vi "FPGAController_v4_slow.vi"() -> ()   [LabVIEW 2013]
uses:
  <vilib>/Utility/miscctls.llb/LVPointTypeDef.ctl
  <userlib>/_OpenG.lib/file/file.llb/Strip Path Extension - Path__ogtk.vi
  <vilib>/FPGAPlugInAG/PXI-7954R/niLvFpga_Open_PXI-7954R.vi
  <userlib>/_OpenG.lib/comparison/comparison.llb/Boolean Changed__ogtk.vi
  <vilib>/addons/database/Connection.llb/Conn Execute.vi
  <vilib>/addons/database/Recordset.llb/Rec Fetch Recordset Data (R).vi
  <vilib>/addons/database/Recordset.llb/Rec Destroy - Connection.vi
  <userlib>/_OpenG.lib/comparison/comparison.llb/DBL Changed__ogtk.vi
  <vilib>/Utility/error.llb/Error Cluster From Error Code.vi
  <vilib>/rvi/errors/niLvFpgaAdjustHostInterfaceError.vi
  <vilib>/FPGAPlugInAG/PXI-7954R/niLvFpga_Close_PXI-7954R.vi
  <vilib>/rvi/interface/nirviOpenFPGA/nirviOpenFPGA.xnode
  FPGA Bitfiles/correlationwithf_FPGATarget_FPGAcodeslow_ywMU-DMuSi0.lvbitx
  <vilib>/addons/database/_DB Variant To Data/Database Variant To Data.xnode
  <vilib>/rvi/interface/nirviMethod/nirviMethod.xnode
  <vilib>/FPGA/interface/niFpgaViExecutionMode.ctl
  <vilib>/rvi/interface/nirviReadWriteControl/nirviReadWriteControl.xnode
  <vilib>/rvi/interface/nirviCloseFPGA/nirviCloseFPGA.xnode
  <vilib>/addons/database/NI_Database_API.lvlib
  NiFpgaLv.dll
panel:
  out "Time Betwee Shots":dbl
  out "Del Armed":bool
  in  "Lower Threshold":bool
  in  "Raise Threshold":bool
  out "Update Threshold":bool
  in  "Min. Time\nBetween Shots (s)":dbl
  in  "Rate Limiting":bool
  out "Armed":bool
  in  "Add Delay":bool
  in  "Delay Name":string
  in  "Delay Value":dbl=3.0 min=0.0
  in  "Delay Ring":dbl(ring)=3.15039 items=["Ablation Chamber"=6.45, "LEIL Chamber"=4.318, "Thid Detector"=3.15039, "Custom"=0.0]
  in  "Rearm Trigger":bool
  in  "One Shot Mode":bool
  out "Last Update:":timestamp
  out "Updating FPGA":bool
  out "Sensitivity":dbl
  out "error out":errorcluster
  out "Low Mass Limit":fxp<+,31,17>
  out "High Mass Limit":fxp<+,31,17>
  out "stopping":bool
  in  "Auto Threshold":bool
  out "Peletron (MV)":dbl=2.0
  out "High Mass (kg)":dbl=inf
  out "Low Mass (kg)":dbl
  out "High Charge Limit":i16
  out "Low Charge Limit":i16
  out "High velocity count":i32=210
  out "Low velocity count":i32=21000
  in  "stop":bool
  in  "Peak-Threshold Factor":dbl=2.0
  out "Low Charge Limit (fC)":dbl
  out "High Charge Limit (fC)":dbl=100.0
  out "High Velocity":dbl=100000.0
  out "Low Velocity":dbl=1000.0
  out "Filter 7 Peak":i32=7483
  out "Filter 6 Peak":i32=9863
  out "Filter 5 Peak":i32=13910
  out "Filter 4 Peak":i32=18191
  out "Filter 3 Peak":i32=46254
  out "Filter 2 Peak":i32=120664
  out "Filter 1 Peak":i32=295996
  in  "Filter7 Threshold":i32=-21165
  in  "Filter6 Threshold":i32=-29358
  in  "Filter5 Threshold":i32=-41730
  in  "Filter4 Threshold":i32=-54306
  in  "Filter3 Threshold":i32=-138762
  in  "Filter2 Threshold":i32=-361992
  in  "Filter1 Threshold":i32=-887988
  in  "Zero Peak Values":bool
  in  "Assign Threshold":bool
  in  "Run Mode":bool
  # "Settings"
  # "Dubugging"
  # "Independent Variable"
  # "Low Vel."
  # "High Vel."
  # "Low Q (fC)"
  # "High Q (fC)"
  # "Plate Control While Loop Counter"
  # "Low Mass (kg)"
  # "High Mass (kg)"
  # "Sens. (V/pC)"
  # "Peletron (MV)"
  # "Current Value of Running Average"
  # "Peak Threshold Factor"
  # "Delay Trigger"
  # "Dist. from 2nd Det. (m)"
  # "Name"
  # "Peak Values"
  # "Peak 1"
  # "Peak 2"
  # "Peak 3"
  # "Peak 4"
  # "Peak 5"
  # "Peak 6"
  # "Peak 7"
  # "Thresholds"
  # "Threshold 1"
  # "Threshold 2"
  # "Threshold 3"
  # "Threshold 4"
  # "Threshold 5"
  # "Threshold 6"
  # "Threshold 7"
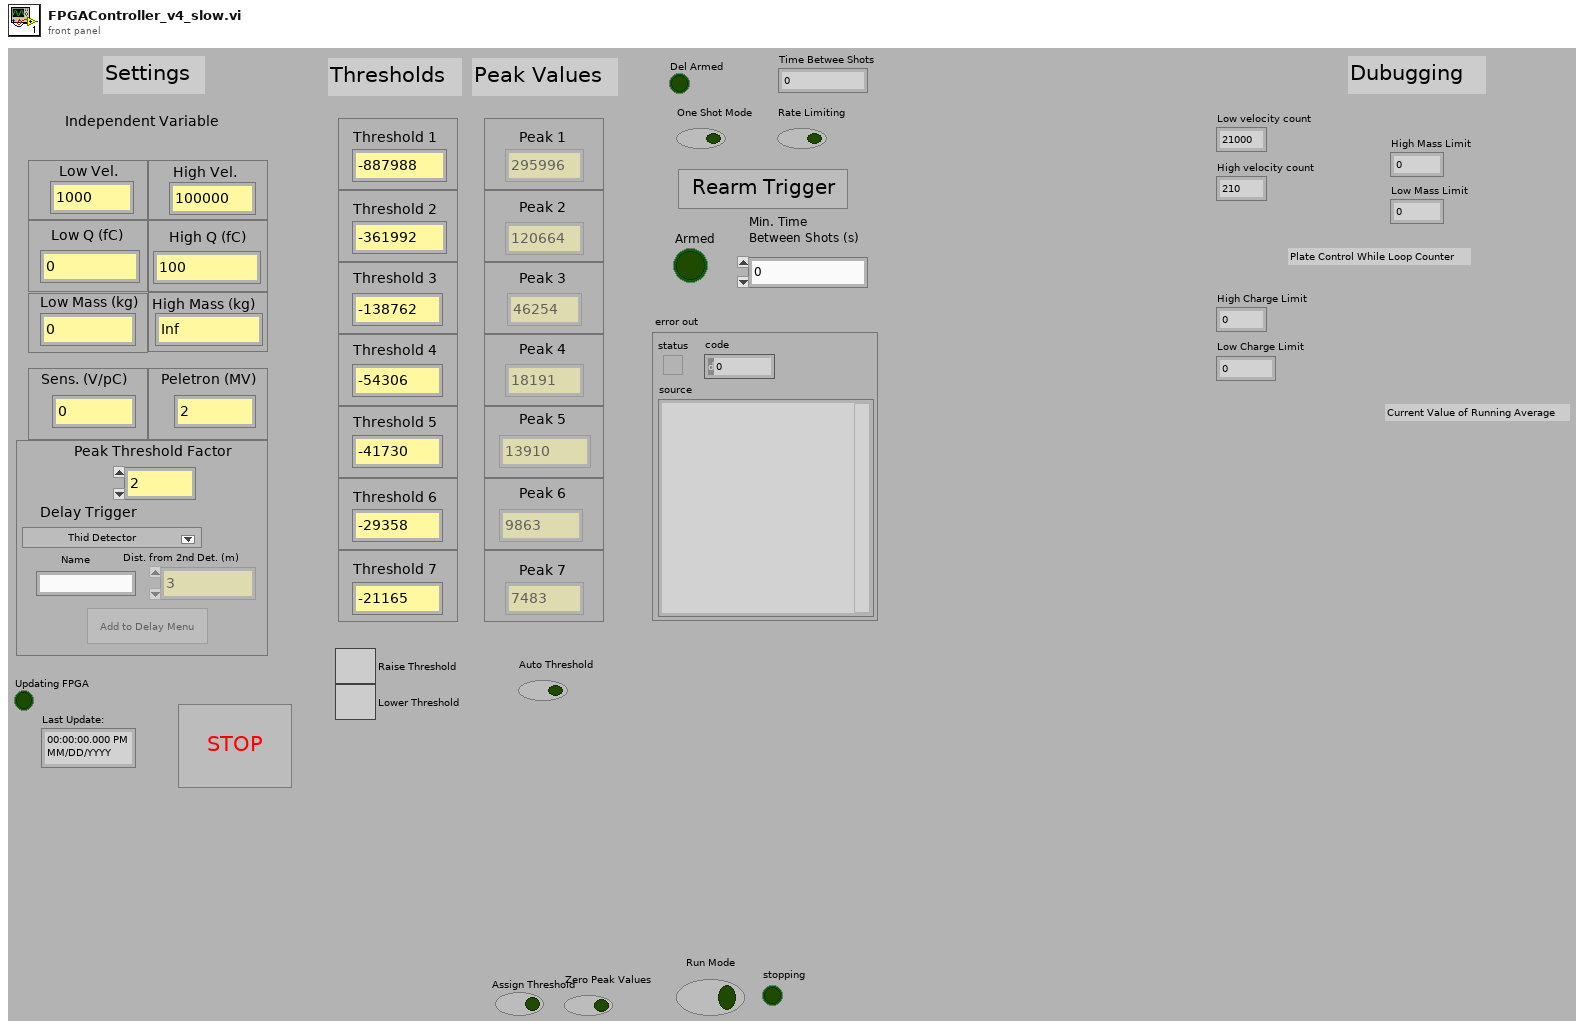
[diagram p1: front panel]
types:
  T1 = typedef "LVPointTypeDef.ctl" = cluster{"Horizontal":i16, "Vertical":i16}
  T2 = enum8{"Enabled", "Disabled", "Disabled and Grayed Out"}
  T3 = typedef "NI_Database_API.lvlib/Conn ObjectReference.ctl" = refnum<k1>
  T4 = cluster{"Filter 1 Peak":i32, "Filter 2 Peak":i32, "Filter 3 Peak":i32, "Filter 4 Peak":i32, "Filter 5 Peak":i32, "Filter 6 Peak":i32, "Filter 7 Peak":i32}
  T5 = typedef "NI_Database_API.lvlib/Rec ObjectReference.ctl" = refnum<k1>
  T6 = typedef "LVStringsAndValuesArrayTypeDef_DBL.ctl" = cluster{"String":string, "Value":dbl}[]
  T7 = cluster{"Numeric":dbl, "Numeric":dbl, "Numeric":dbl, "Numeric":dbl, "Numeric":dbl, "Numeric":dbl, dbl, dbl, "Value":dbl, fxp<+,16,7>, bool}
  T8 = cluster{"Low Velocity Count":i32, "High Velocity Count":i32, "Low Charge Limit (ADC ticks)":i16, "High Charge Limit (ADC ticks)":i16, "Low Mass (ADC*cycle^2)":i64, "High Mass (ADC*cycle^2)":i64, "Mult":fxp<+,16,7>, "Mult Use?":bool}
  T9 = cluster{"Filter 1 Detector 3 Correlation":i32, "Filter 2 Detector 3 Correlation":i32, "Filter 3 Detector 3 Correlation":i32, "Filter 4 Detector 3 Correlation":i32, "Filter 5 Detector 3 Correlation":i32, "Filter 6 Detector 3 Correlation":i32, "Filter 7 Detector 3 Correlation":i32}
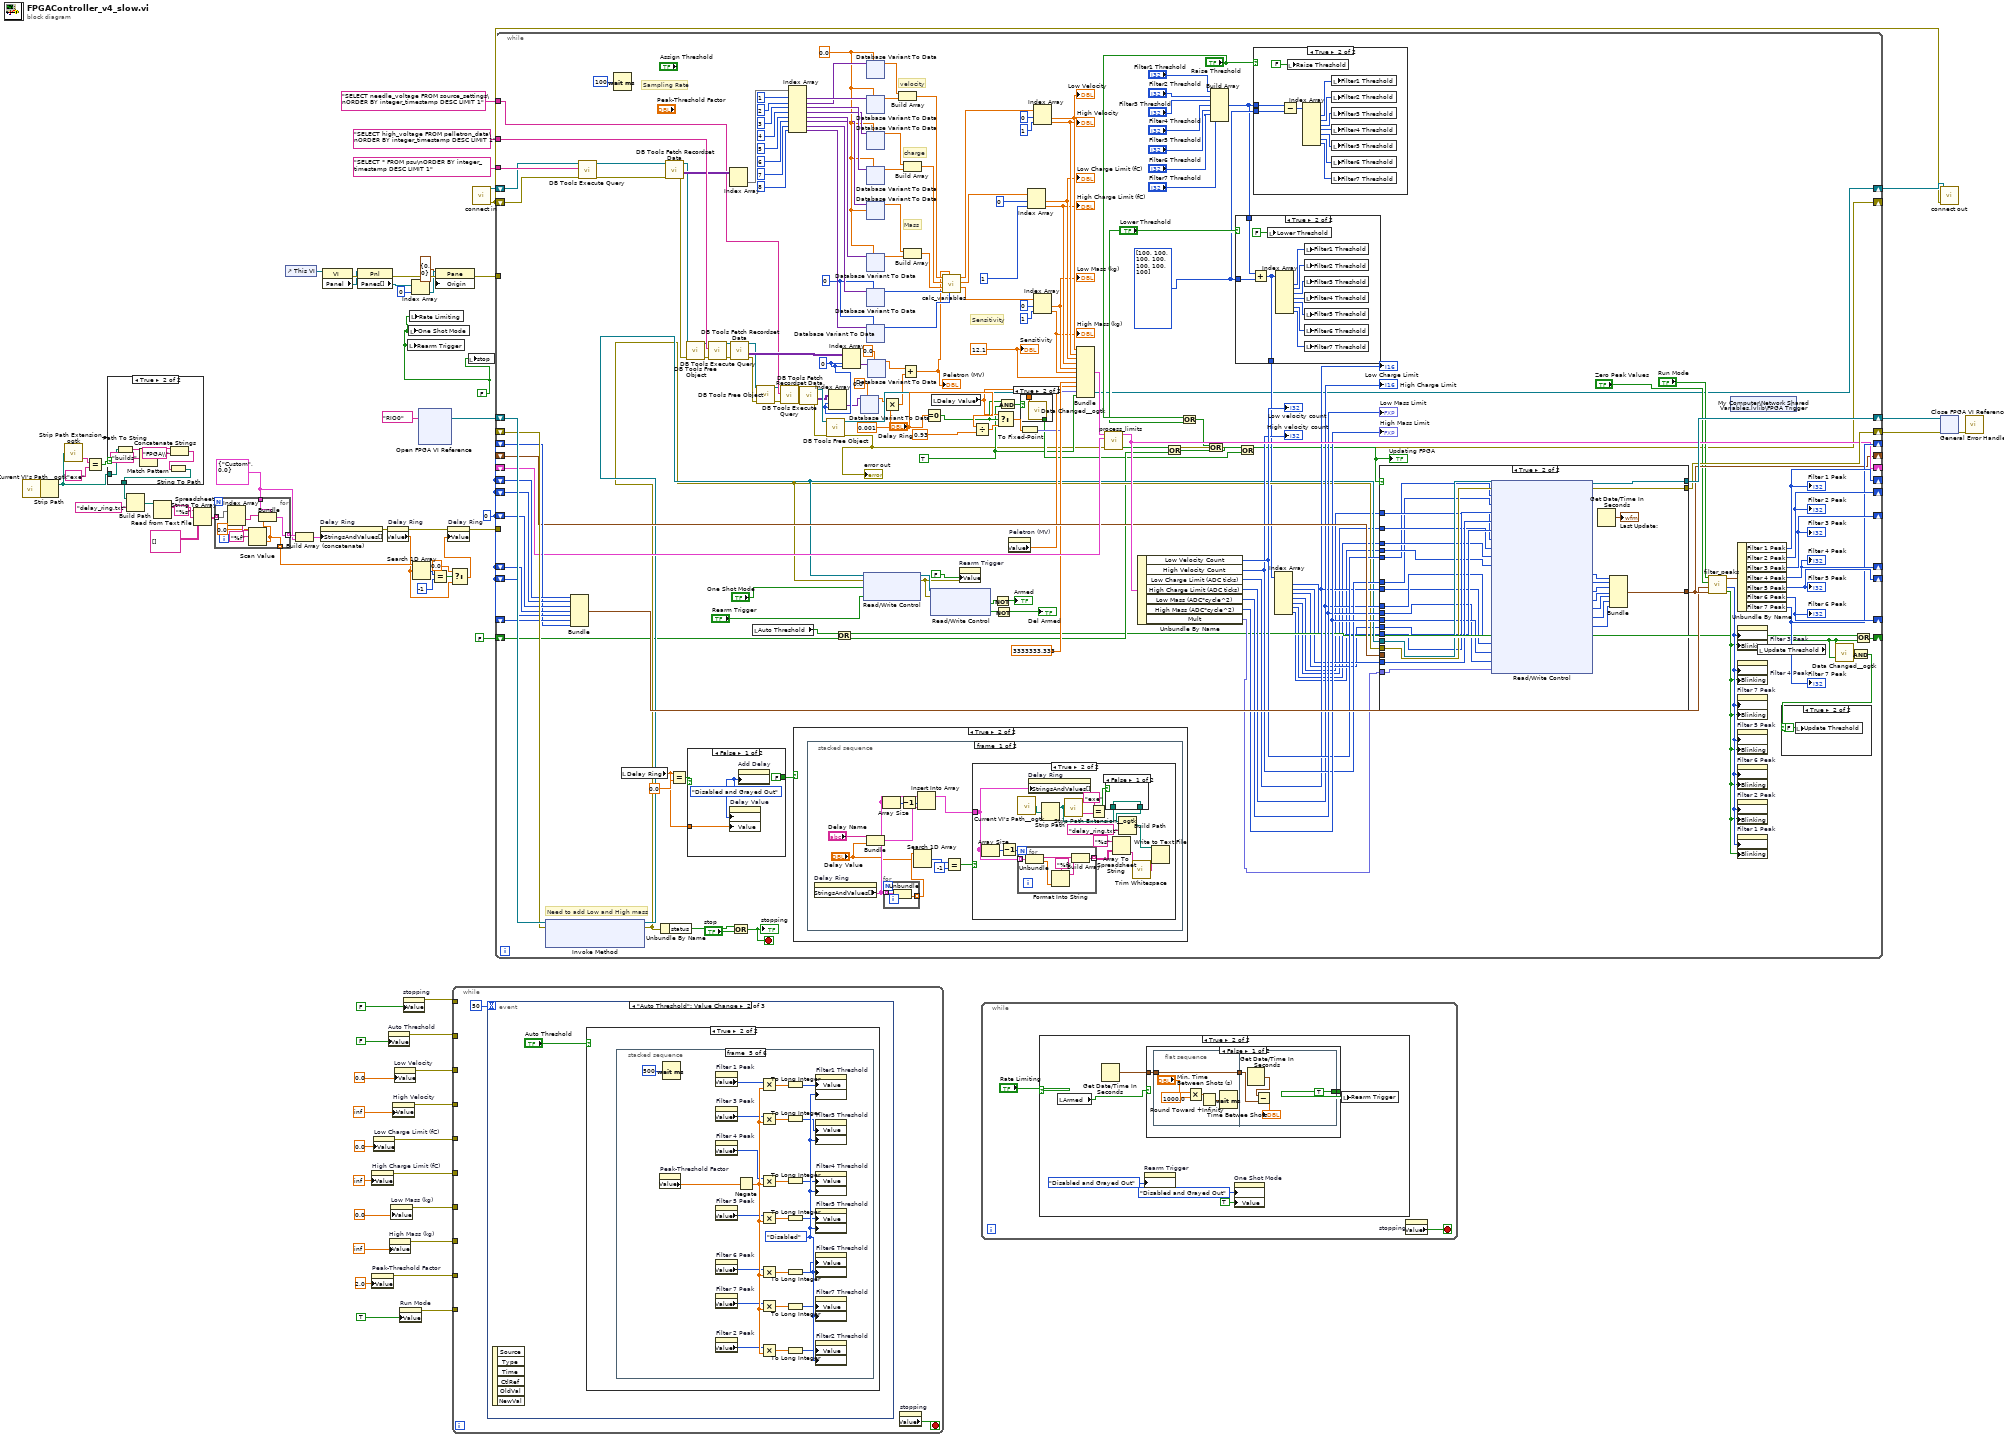
[diagram p0: block diagram]
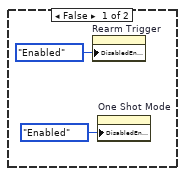
[diagram p3: hidden frame]
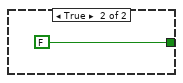
[diagram p4: hidden frame]
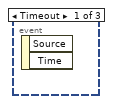
[diagram p5: hidden frame]
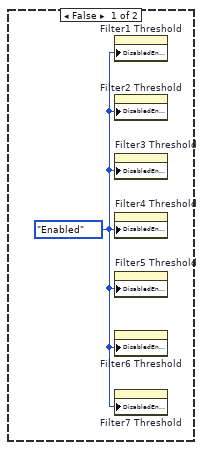
[diagram p6: hidden frame]
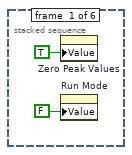
[diagram p7: hidden frame]
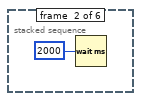
[diagram p8: hidden frame]
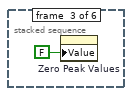
[diagram p9: hidden frame]
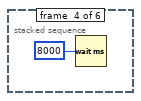
[diagram p10: hidden frame]
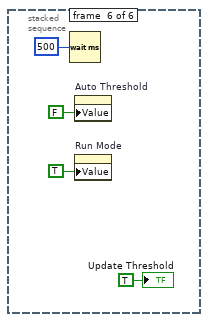
[diagram p11: hidden frame]
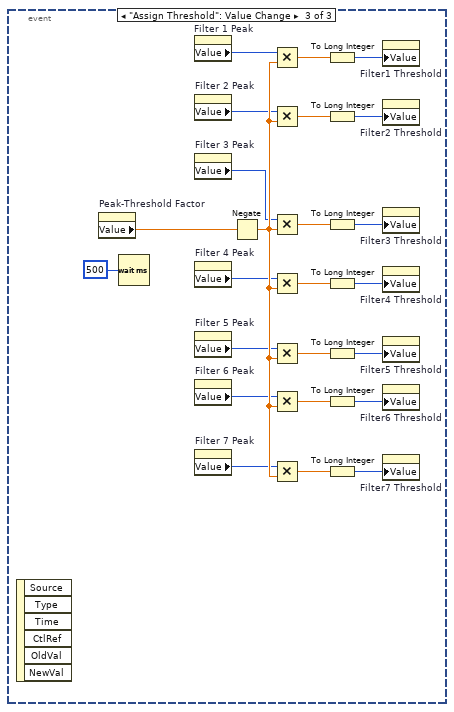
[diagram p12: hidden frame]
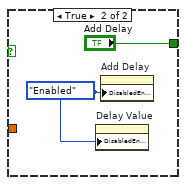
[diagram p17: hidden frame]
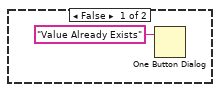
[diagram p19: hidden frame]
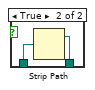
[diagram p20: hidden frame]
diagram:
  w18 = cluster{"String":string, "Value":dbl} {"String"="Custom", "Value"=0.0}
  w28 = FALSE
  w67 = 0
  n1 = call <userlib>:"Current VI's Path__ogtk.vi"() -> ("Current VI's Path (+ Relative)"=w27:path)  [unwired: 1 in]
  n2 = Strip Path(path=w27) -> (stripped path=w13:path)  [unwired: 1 out]
  n3 = call-poly <userlib>:"Strip Path Extension__ogtk.vi"("path"=w13) -> ("extension"=w17:string)  [unwired: 1 out]
  n4 = Equal?(x=w17, y="exe") -> (x = y?=w14:bool)
  n5 = case shown="True" w14 {
    tunnel: w13 -> [w69 w76]
    tunnel: [w69 w70] -> w12
    frame False {
    }
    frame True {
      n6 = Path To String(path=w76) -> (string=w75:string)
      n7 = Match Pattern(string=w75, regular expression="builds") -> (before substring=w73:string)  [unwired: 1 in, 3 out]
      n8 = Concatenate Strings(w73, "FPGA\\" ("string")) -> (w71:string)
      n9 = String To Path(string=w71) -> (path=w70:path)
    }
  }
  n10 = Build Path(base path=w12, name or relative path="delay_ring.txt") -> (appended path=w15:path)
  n11 = Read from Text File(file (use dialog)=w15) -> (text=w25:string)  [unwired: 3 in, 3 out]
  n12 = Spreadsheet String To Array(format string="%s", spreadsheet string=w25, array type (2D Dbl)=string[][] []) -> (array=w22:string[][])  [unwired: 1 in]
  n13 = for {
    tunnel: w22 -> [w84] mode=indexing
    tunnel: w18 -> [w82]
    tunnel: [w78] -> w19 mode=indexing
    tunnel: [w77] -> w11 mode=indexing
    n14 = Index Array(array=w84) -> (element #1=w83:string, element #2=w81:string)  [unwired: 2 in]
    n15 = Scan Value(string=w81, format string="%f", default (0 dbl)=0.0) -> (value=w77:dbl)  [unwired: 1 out]
    n16 = Bundle(cluster=w82, "String"=w83, "Value"=w77) -> (w78:cluster{"String":string, "Value":dbl})
  }
  n17 = control-ref of="This VI"() -> (w39:refnum<vi>)
  n18 = Build Array (concatenate)(w19, w18) -> (w21:cluster{"String":string, "Value":dbl}[])
  n19 = property on="Delay Ring" class="Ring (strict)"("StringsAndValues[]"=w21) -> (error out=w20:errorcluster)  [unwired: 2 in, 1 out]
  n20 = property class="VI"(reference=w39) -> (error out=w38:errorcluster, "Panel"=w37:refnum<vi>)  [unwired: 1 in, 1 out]
  n21 = property class="Pnl"(reference=w37, error in=w38) -> (error out=w36:errorcluster, "Panes[]"=w35:refnum<vi>[])  [unwired: 1 out]
  n22 = property on="High Charge Limit (fC)" class="DigNum (strict)"("Value"=inf ("High Charge Limit (fC)")) -> (error out=w54:errorcluster)  [unwired: 2 in, 1 out]
  n23 = property on="Peak-Threshold Factor" class="DigNum (strict)"("Value"=2.0 ("Peak-Threshold Factor")) -> (error out=w48:errorcluster)  [unwired: 2 in, 1 out]
  n24 = property on="Low Charge Limit (fC)" class="DigNum (strict)"("Value"=0.0 ("Low Charge Limit (fC)")) -> (error out=w56:errorcluster)  [unwired: 2 in, 1 out]
  n25 = property on="Delay Ring" class="Ring (strict)"(error in=w20) -> (error out=w10:errorcluster, "Value"=w4:dbl)  [unwired: 1 in, 1 out]
  n26 = property on="Auto Threshold" class="Bool (strict)"("Value"=FALSE ("Auto Threshold")) -> (error out=w62:errorcluster)  [unwired: 2 in, 1 out]
  n27 = property on="High Mass (kg)" class="DigNum (strict)"("Value"=inf ("High Mass (kg)")) -> (error out=w50:errorcluster)  [unwired: 2 in, 1 out]
  n28 = property on="Low Mass (kg)" class="DigNum (strict)"("Value"=0.0 ("Low Mass (kg)")) -> (error out=w52:errorcluster)  [unwired: 2 in, 1 out]
  n29 = property on="High Velocity" class="DigNum (strict)"("Value"=inf ("High Velocity")) -> (error out=w58:errorcluster)  [unwired: 2 in, 1 out]
  n30 = property on="Low Velocity" class="DigNum (strict)"("Value"=0.0 ("Low Velocity")) -> (error out=w60:errorcluster)  [unwired: 2 in, 1 out]
  n31 = property on="Run Mode" class="Bool (strict)"("Value"=TRUE ("Run Mode")) -> (error out=w46:errorcluster)  [unwired: 2 in, 1 out]
  n32 = property on="stopping" class="Bool (strict)"("Value"=FALSE ("stopping")) -> (error out=w64:errorcluster)  [unwired: 2 in, 1 out]
  n33 = local write "Rearm Trigger"(w28) -> ()
  n34 = local write "One Shot Mode"(w28) -> ()
  n35 = local write "Rate Limiting"(w28) -> ()
  n36 = Index Array(array=w35, index=0) -> (element=w33:refnum<vi>)
  n37 = Search 1D Array(1D array=w11, element=w4) -> (index of element=w8:i32)  [unwired: 1 in]
  n38 = xnode "Open FPGA VI Reference"("resource name"=tag "RIO0") -> ("FPGA VI Reference Out"=w30:refnum<k20>)  [unwired: 1 in, 1 out]
  n39 = Equal?(x=w8, y=-1) -> (x = y?=w6:bool)
  n40 = property class="Pane"(reference=w33, error in=w36, "Origin"=T1 {"Horizontal"=0, "Vertical"=0}) -> (error out=w31:errorcluster)  [unwired: 1 out]
  n41 = Select(t=0.0, s=w6, f=w4) -> (s? t:f=w5:dbl)
  n42 = property on="Delay Ring" class="Ring (strict)"(error in=w10, "Value"=w5) -> (error out=w9:errorcluster)  [unwired: 1 in, 1 out]
  n43 = while {
    tunnel: w64 -> [_]
    tunnel: w62 -> [_]
    tunnel: w60 -> [_]
    tunnel: w58 -> [_]
    tunnel: w56 -> [_]
    tunnel: w54 -> [_]
    tunnel: w52 -> [_]
    tunnel: w50 -> [_]
    tunnel: w48 -> [_]
    tunnel: w46 -> [_]
    stop <- w86 stop-if-true
    n44 = event shown="[1] \"Auto Threshold\": Value Change" {
      selector: _ -> [_ _ _]
      dyn-events: _ -> [_ _ _]
      timeout: 50 -> [_ _ _]
      event Timeout {
        n45 = event-data() -> ()  [unwired: 1 in, 2 out]
      }
      event "Auto Threshold": Value Change {
        n46 = event-data() -> ()  [unwired: 1 in, 6 out]
        n47 = case shown="True" "Auto Threshold" {
          frame False {
            w88 = T2."Enabled" ("Disabled")
            n48 = property on="Filter1 Threshold" class="DigNum (strict)"("DisabledEnum"=w88) -> ()  [unwired: 2 in, 2 out]
            n49 = property on="Filter2 Threshold" class="DigNum (strict)"("DisabledEnum"=w88) -> ()  [unwired: 2 in, 2 out]
            n50 = property on="Filter3 Threshold" class="DigNum (strict)"("DisabledEnum"=w88) -> ()  [unwired: 2 in, 2 out]
            n51 = property on="Filter4 Threshold" class="DigNum (strict)"("DisabledEnum"=w88) -> ()  [unwired: 2 in, 2 out]
            n52 = property on="Filter5 Threshold" class="DigNum (strict)"("DisabledEnum"=w88) -> ()  [unwired: 2 in, 2 out]
            n53 = property on="Filter6 Threshold" class="DigNum (strict)"("DisabledEnum"=w88) -> ()  [unwired: 2 in, 2 out]
            n54 = property on="Filter7 Threshold" class="DigNum (strict)"("DisabledEnum"=w88) -> ()  [unwired: 2 in, 2 out]
          }
          frame True {
            n55 = stacked-sequence {
              frame #0 {
                n56 = property on="Zero Peak Values" class="Bool (strict)"("Value"=TRUE ("Zero Peak Values")) -> ()  [unwired: 2 in, 2 out]
                n57 = property on="Run Mode" class="Bool (strict)"("Value"=FALSE ("Run Mode")) -> ()  [unwired: 2 in, 2 out]
              }
              frame #1 {
                n58 = Wait (ms)(milliseconds to wait=u32 2000) -> ()  [unwired: 1 out]
              }
              frame #2 {
                n59 = property on="Zero Peak Values" class="Bool (strict)"("Value"=FALSE ("Zero Peak Values")) -> ()  [unwired: 2 in, 2 out]
              }
              frame #3 {
                n60 = Wait (ms)(milliseconds to wait=u32 8000) -> ()  [unwired: 1 out]
              }
              frame #4 {
                w118 = T2."Disabled" ("Disabled")
                n61 = property on="Peak-Threshold Factor" class="DigNum (strict)"() -> ("Value"=w103:dbl)  [unwired: 2 in, 2 out]
                n62 = Wait (ms)(milliseconds to wait=u32 500) -> ()  [unwired: 1 out]
                n63 = property on="Filter 1 Peak" class="DigNum (strict)"() -> ("Value"=w101:i32)  [unwired: 2 in, 2 out]
                n64 = property on="Filter 3 Peak" class="DigNum (strict)"() -> ("Value"=w99:i32)  [unwired: 2 in, 2 out]
                n65 = property on="Filter 4 Peak" class="DigNum (strict)"() -> ("Value"=w98:i32)  [unwired: 2 in, 2 out]
                n66 = property on="Filter 5 Peak" class="DigNum (strict)"() -> ("Value"=w97:i32)  [unwired: 2 in, 2 out]
                n67 = property on="Filter 6 Peak" class="DigNum (strict)"() -> ("Value"=w96:i32)  [unwired: 2 in, 2 out]
                n68 = property on="Filter 7 Peak" class="DigNum (strict)"() -> ("Value"=w95:i32)  [unwired: 2 in, 2 out]
                n69 = property on="Filter 2 Peak" class="DigNum (strict)"() -> ("Value"=w100:i32)  [unwired: 2 in, 2 out]
                n70 = Negate(x=w103) -> (-x=w102:dbl)
                n71 = Multiply(x=w101, y=w102) -> (x*y=w117:dbl)
                n72 = Multiply(x=w99, y=w102) -> (x*y=w113:dbl)
                n73 = Multiply(x=w98, y=w102) -> (x*y=w111:dbl)
                n74 = Multiply(x=w97, y=w102) -> (x*y=w109:dbl)
                n75 = Multiply(x=w96, y=w102) -> (x*y=w107:dbl)
                n76 = Multiply(x=w95, y=w102) -> (x*y=w105:dbl)
                n77 = Multiply(x=w100, y=w102) -> (x*y=w115:dbl)
                n78 = To Long Integer(number=w117) -> (32bit integer=w116:i32)
                n79 = To Long Integer(number=w113) -> (32bit integer=w112:i32)
                n80 = To Long Integer(number=w111) -> (32bit integer=w110:i32)
                n81 = To Long Integer(number=w109) -> (32bit integer=w108:i32)
                n82 = To Long Integer(number=w107) -> (32bit integer=w106:i32)
                n83 = To Long Integer(number=w105) -> (32bit integer=w104:i32)
                n84 = To Long Integer(number=w115) -> (32bit integer=w114:i32)
                n85 = property on="Filter1 Threshold" class="DigNum (strict)"("Value"=w116, "DisabledEnum"=w118) -> ()  [unwired: 2 in, 2 out]
                n86 = property on="Filter3 Threshold" class="DigNum (strict)"("Value"=w112, "DisabledEnum"=w118) -> ()  [unwired: 2 in, 2 out]
                n87 = property on="Filter4 Threshold" class="DigNum (strict)"("Value"=w110, "DisabledEnum"=w118) -> ()  [unwired: 2 in, 2 out]
                n88 = property on="Filter5 Threshold" class="DigNum (strict)"("Value"=w108, "DisabledEnum"=w118) -> ()  [unwired: 2 in, 2 out]
                n89 = property on="Filter6 Threshold" class="DigNum (strict)"("Value"=w106, "DisabledEnum"=w118) -> ()  [unwired: 2 in, 2 out]
                n90 = property on="Filter7 Threshold" class="DigNum (strict)"("Value"=w104, "DisabledEnum"=w118) -> ()  [unwired: 2 in, 2 out]
                n91 = property on="Filter2 Threshold" class="DigNum (strict)"("Value"=w114, "DisabledEnum"=w118) -> ()  [unwired: 2 in, 2 out]
              }
              frame #5 {
                n92 = Wait (ms)(milliseconds to wait=u32 500) -> ()  [unwired: 1 out]
                n93 = property on="Auto Threshold" class="Bool (strict)"("Value"=FALSE ("Auto Threshold")) -> ()  [unwired: 2 in, 2 out]
                n94 = property on="Run Mode" class="Bool (strict)"("Value"=TRUE ("Run Mode")) -> ()  [unwired: 2 in, 2 out]
                "Update Threshold" <- TRUE ("Update Threshold")
              }
            }
          }
        }
      }
      event "Assign Threshold": Value Change {
        n95 = event-data() -> ()  [unwired: 1 in, 6 out]
        n96 = property on="Peak-Threshold Factor" class="DigNum (strict)"() -> ("Value"=w137:dbl)  [unwired: 2 in, 2 out]
        n97 = Wait (ms)(milliseconds to wait=u32 500) -> ()  [unwired: 1 out]
        n98 = property on="Filter 1 Peak" class="DigNum (strict)"() -> ("Value"=w136:i32)  [unwired: 2 in, 2 out]
        n99 = property on="Filter 2 Peak" class="DigNum (strict)"() -> ("Value"=w135:i32)  [unwired: 2 in, 2 out]
        n100 = property on="Filter 3 Peak" class="DigNum (strict)"() -> ("Value"=w134:i32)  [unwired: 2 in, 2 out]
        n101 = property on="Filter 4 Peak" class="DigNum (strict)"() -> ("Value"=w133:i32)  [unwired: 2 in, 2 out]
        n102 = property on="Filter 5 Peak" class="DigNum (strict)"() -> ("Value"=w132:i32)  [unwired: 2 in, 2 out]
        n103 = property on="Filter 6 Peak" class="DigNum (strict)"() -> ("Value"=w131:i32)  [unwired: 2 in, 2 out]
        n104 = property on="Filter 7 Peak" class="DigNum (strict)"() -> ("Value"=w130:i32)  [unwired: 2 in, 2 out]
        n105 = Negate(x=w137) -> (-x=w139:dbl)
        n106 = Multiply(x=w136, y=w139) -> (x*y=w146:dbl)
        n107 = Multiply(x=w135, y=w139) -> (x*y=w144:dbl)
        n108 = Multiply(x=w134, y=w139) -> (x*y=w143:dbl)
        n109 = Multiply(x=w133, y=w139) -> (x*y=w142:dbl)
        n110 = Multiply(x=w132, y=w139) -> (x*y=w141:dbl)
        n111 = Multiply(x=w131, y=w139) -> (x*y=w140:dbl)
        n112 = Multiply(x=w130, y=w139) -> (x*y=w145:dbl)
        n113 = To Long Integer(number=w146) -> (32bit integer=w129:i32)
        n114 = To Long Integer(number=w144) -> (32bit integer=w128:i32)
        n115 = To Long Integer(number=w143) -> (32bit integer=w127:i32)
        n116 = To Long Integer(number=w142) -> (32bit integer=w126:i32)
        n117 = To Long Integer(number=w141) -> (32bit integer=w125:i32)
        n118 = To Long Integer(number=w140) -> (32bit integer=w124:i32)
        n119 = To Long Integer(number=w145) -> (32bit integer=w123:i32)
        n120 = property on="Filter1 Threshold" class="DigNum (strict)"("Value"=w129) -> ()  [unwired: 2 in, 2 out]
        n121 = property on="Filter2 Threshold" class="DigNum (strict)"("Value"=w128) -> ()  [unwired: 2 in, 2 out]
        n122 = property on="Filter3 Threshold" class="DigNum (strict)"("Value"=w127) -> ()  [unwired: 2 in, 2 out]
        n123 = property on="Filter4 Threshold" class="DigNum (strict)"("Value"=w126) -> ()  [unwired: 2 in, 2 out]
        n124 = property on="Filter5 Threshold" class="DigNum (strict)"("Value"=w125) -> ()  [unwired: 2 in, 2 out]
        n125 = property on="Filter6 Threshold" class="DigNum (strict)"("Value"=w124) -> ()  [unwired: 2 in, 2 out]
        n126 = property on="Filter7 Threshold" class="DigNum (strict)"("Value"=w123) -> ()  [unwired: 2 in, 2 out]
      }
    }
    n127 = property on="stopping" class="Bool (strict)"() -> ("Value"=w86:bool)  [unwired: 2 in, 2 out]
  }
  n128 = local write "stop"(w28) -> ()
  n129 = call "connect in.vi"() -> ("error out"=w40:errorcluster, "Database Connection"=w41:T3)  [unwired: 7 in, 1 out]
  n130 = while {
    shift-right: [w322] -> w66
    shift-left: w30 -> [w326]
    shift-right: [w321] -> w65
    shift-left: _ -> [w325]
    shift-right: [w317] -> _
    shift-left: w67 -> [w310]
    shift-right: [w316] -> _
    shift-left: w67 -> [w309]
    shift-right: [w315] -> _
    shift-left: w67 -> [w308]
    shift-right: [w314] -> _
    shift-left: w67 -> [w307]
    shift-right: [w313] -> _
    shift-left: w67 -> [w306]
    shift-right: [w319] -> _
    shift-left: w67 -> [w312]
    shift-right: [w318] -> _
    shift-left: w67 -> [w311]
    tunnel: "SELECT * FROM psu\nORDER BY integer_timestamp DESC LIMIT 1" ("SQL query") -> [w305]
    tunnel: "SELECT high_voltage FROM pelletron_data\nORDER BY integer_timestamp DESC LIMIT 1" ("SQL query") -> [w304]
    shift-right: [w156] -> w42
    shift-left: w41 -> [w303]
    shift-right: [w157] -> _
    shift-left: w40 -> [w302]
    shift-right: [w301] -> _
    shift-left: _ -> [w300]
    shift-right: [w298] -> _
    shift-left: _ -> [w299]
    tunnel: w31 -> [_]
    tunnel: w9 -> [_]
    shift-right: [w203] -> _
    shift-left: FALSE -> [w206]
    tunnel: "SELECT needle_voltage FROM source_settings\nORDER BY integer_timestamp DESC LIMIT 1" ("SQL query") -> [w164]
    stop <- w320 stop-if-true
    w166 = i32[] [100, 100, 100, 100, 100, 100, 100]
    w169 = TRUE
    w154 = 0 ("index (row)")
    w262 = i8 0
    w263 = 0.0
    w229 = 12.1
    # "charge"
    # "Mass"
    # "velocity"
    # "Sensitivity"
    # "Sampling Rate"
    # "Need to add Low and High mass"
    n131 = xnode "Invoke Method"("FPGA VI Reference In"=w326, "error in"=w325) -> ("FPGA VI Reference Out"=w223:refnum<k20>, "error out"=w222:errorcluster)  [unwired: 1 out]
    n132 = Bundle("Filter 1 Peak"=w312, "Filter 2 Peak"=w311, "Filter 3 Peak"=w310, "Filter 4 Peak"=w309, "Filter 5 Peak"=w308, "Filter 6 Peak"=w307, "Filter 7 Peak"=w306) -> (w294:T4)  [unwired: 1 in]
    n133 = call-poly <vilib>:"DB Tools Execute Query.vi"("error in (no error)"=w302, "SQL query"=w305, "connection reference"=w303) -> ("error out"=w282:errorcluster, "recordset reference"=w283:T5)  [unwired: 5 in]
    n134 = Wait (ms)(milliseconds to wait=u32 100) -> ()  [unwired: 1 out]
    n135 = local read "Delay Ring"() -> (w207:dbl)
    n136 = Unbundle By Name(w222) -> ("status"=w324:bool)
    n137 = call-poly <vilib>:"DB Tools Fetch Recordset Data.vi"("error in (no error)"=w282, "recordset reference"=w283) -> ("error out"=w260:errorcluster, "recordset data"=w273:variant[][], "recordset reference out"=w261:T5)  [unwired: 3 in]
    n138 = Equal?(x=w207, y=0.0) -> (x = y?=w208:bool)
    n139 = call-poly <vilib>:"DB Tools Free Object.vi"("error in (no error)"=w260, "recordset reference"=w261) -> ("error out"=w258:errorcluster, "connection reference"=w259:T3)  [unwired: 8 in]
    n140 = case shown="False" w208 {
      tunnel: [FALSE ("Add Delay") "Add Delay"] -> w226
      tunnel: w207 -> [w387 _]
      frame False {
        w388 = T2."Disabled and Grayed Out" ("Disabled")
        n141 = property on="Delay Value" class="DigNum (strict)"("DisabledEnum"=w388, "Value"=w387) -> ()  [unwired: 2 in, 2 out]
        n142 = property on="Add Delay" class="Bool (strict)"("DisabledEnum"=w388) -> ()  [unwired: 2 in, 2 out]
      }
      frame True {
        w389 = T2."Enabled" ("Disabled")
        n143 = property on="Delay Value" class="DigNum (strict)"("DisabledEnum"=w389) -> ()  [unwired: 2 in, 2 out]
        n144 = property on="Add Delay" class="Bool (strict)"("DisabledEnum"=w389) -> ()  [unwired: 2 in, 2 out]
      }
    }
    n145 = call-poly <vilib>:"DB Tools Execute Query.vi"("error in (no error)"=w258, "SQL query"=w304, "connection reference"=w259) -> ("error out"=w256:errorcluster, "recordset reference"=w257:T5)  [unwired: 5 in]
    n146 = Index Array(array=w273) -> (element=w272:variant[])  [unwired: 2 in]
    n147 = call-poly <vilib>:"DB Tools Fetch Recordset Data.vi"("error in (no error)"=w256, "recordset reference"=w257) -> ("error out"=w230:errorcluster, "recordset data"=w255:variant[][], "recordset reference out"=w231:T5)  [unwired: 3 in]
    n148 = Or(x=w324, y="stop") -> (x .or. y?=w320:bool)
    "stopping" <- w320
    n149 = local read "Auto Threshold"() -> (w204:bool)
    n150 = call-poly <vilib>:"DB Tools Free Object.vi"("error in (no error)"=w230, "recordset reference"=w231) -> ("error out"=w162:errorcluster, "connection reference"=w163:T3)  [unwired: 8 in]
    n151 = call-poly <vilib>:"DB Tools Execute Query.vi"("error in (no error)"=w162, "SQL query"=w164, "connection reference"=w163) -> ("error out"=w160:errorcluster, "recordset reference"=w161:T5)  [unwired: 5 in]
    n152 = Index Array(array=w272, index #1=1 ("index"), index #2=2 ("index"), index #3=3 ("index"), index #4=4 ("index"), index #5=5 ("index"), index #6=6 ("index"), index #7=7 ("index"), index #8=8 ("index")) -> (element #1=w271:variant, element #2=w270:variant, element #3=w269:variant, element #4=w268:variant, element #5=w267:variant, element #6=w266:variant, element #7=w265:variant, element #8=w264:variant)
    n153 = case shown="True" w226 {
      frame False {
      }
      frame True {
        n154 = stacked-sequence {
          frame #0 {
            n155 = property on="Delay Ring" class="Ring (strict)"() -> ("StringsAndValues[]"=w393:T6)  [unwired: 2 in, 2 out]
            n156 = Bundle("Delay Name"="Delay Name", "Delay Value"="Delay Value") -> (w398:cluster{"Delay Name":string, "Delay Value":dbl})  [unwired: 1 in]
            n157 = Array Size(array=w393) -> (size(s)=w396:i32)
            n158 = for {
              tunnel: w393 -> [w403] mode=indexing
              tunnel: [w402] -> w392 mode=indexing
              n159 = Unbundle(w403) -> ("Value"=w402:dbl)  [unwired: 1 out]
            }
            n160 = Decrement(x=w396) -> (x-1=w395:i32)
            n161 = Search 1D Array(1D array=w392, element="Delay Value") -> (index of element=w400:i32)  [unwired: 1 in]
            n162 = Insert Into Array(array=w393, index=w395, new element=w398) -> (w397:T6)
            n163 = Equal?(x=w400, y=-1) -> (x = y?=w394:bool)
            n164 = case shown="True" w394 {
              tunnel: w397 -> [_ w412]
              frame False {
                n165 = One Button Dialog(message="Value Already Exists") -> ()  [unwired: 1 in, 1 out]
              }
              frame True {
                n166 = Array Size(array=w412) -> (size(s)=w414:i32)
                n167 = Decrement(x=w414) -> (x-1=w413:i32)
                n168 = call <userlib>:"Current VI's Path__ogtk.vi"() -> ("Current VI's Path (+ Relative)"=w418:path)  [unwired: 1 in]
                n169 = for {
                  N: w413 -> [_]
                  tunnel: w412 -> [w428] mode=indexing
                  tunnel: [w423] -> w415 mode=indexing
                  n170 = Unbundle(w428) -> ("String"=w424:string, "Value"=w427:dbl)
                  n171 = Format Into String(format string="%f", w427) -> (resulting string=w425:string)  [unwired: 2 in, 1 out]
                  n172 = Build Array(w424, w425) -> (w423:string[])
                }
                n173 = property on="Delay Ring" class="Ring (strict)"("StringsAndValues[]"=w412) -> ()  [unwired: 2 in, 2 out]
                n174 = Strip Path(path=w418) -> (stripped path=w406:path)  [unwired: 1 out]
                n175 = call-poly <userlib>:"Strip Path Extension__ogtk.vi"("path"=w406) -> ("extension"=w409:string)  [unwired: 1 out]
                n176 = Equal?(x="exe", y=w409) -> (x = y?=w407:bool)
                n177 = case shown="False" w407 {
                  tunnel: w406 -> [w420 w422]
                  tunnel: [w420 w421] -> w405
                  frame False {
                  }
                  frame True {
                    n178 = Strip Path(path=w422) -> (stripped path=w421:path)  [unwired: 1 out]
                  }
                }
                n179 = Array To Spreadsheet String(array=w415, 3:"%s" ("format string")) -> (spreadsheet string=w411:string)  [unwired: 1 in]
                n180 = Build Path(base path=w405, name or relative path="delay_ring.txt") -> (appended path=w416:path)
                n181 = call <vilib>:"Trim Whitespace.vi"("string"=w411) -> ("trimmed string"=w410:string)  [unwired: 1 in]
                n182 = Write to Text File(file (use dialog)=w416, text=w410) -> ()  [unwired: 2 in, 3 out]
              }
            }
          }
          frame #1 {
            n183 = property on="Add Delay" class="Bool (strict)"("Value"=FALSE ("Add Delay")) -> ()  [unwired: 2 in, 2 out]
          }
        }
      }
    }
    n184 = call-poly <vilib>:"DB Tools Fetch Recordset Data.vi"("error in (no error)"=w160, "recordset reference"=w161) -> ("error out"=w158:errorcluster, "recordset data"=w155:variant[][], "recordset reference out"=w159:T5)  [unwired: 3 in]
    n185 = call-poly <vilib>:"DB Tools Free Object.vi"("error in (no error)"=w158, "recordset reference"=w159) -> ("error out"=w157:errorcluster, "connection reference"=w156:T3)  [unwired: 8 in]
    "error out" <- w157
    n186 = Index Array(array=w155, index (row)=w154, index (col)=w154) -> (element=w153:variant)
    n187 = Or(x=w204, y=w206) -> (x .or. y?=w205:bool)
    n188 = Index Array(array=w255, index (row)=w154, index (col)=w154) -> (element=w254:variant)
    n189 = xnode "Database Variant To Data"("database variant"=w153, "type"=0.0) -> ("data"=w151:dbl)  [unwired: 1 in, 1 out]
    n190 = xnode "Read/Write Control"("FPGA VI Reference In"=w223, "error in"=w222, "One Shot"="One Shot Mode", "Reset One Shot"="Rearm Trigger") -> ("FPGA VI Reference Out"=w216:refnum<k20>, "error out"=w215:errorcluster)
    n191 = xnode "Database Variant To Data"("database variant"=w270, "type"=w263) -> ("data"=w179:dbl)  [unwired: 1 in, 1 out]
    n192 = xnode "Database Variant To Data"("database variant"=w271, "type"=w263) -> ("data"=w180:dbl)  [unwired: 1 in, 1 out]
    n193 = xnode "Database Variant To Data"("database variant"=w268, "type"=w263) -> ("data"=w178:dbl)  [unwired: 1 in, 1 out]
    n194 = xnode "Database Variant To Data"("database variant"=w269, "type"=w263) -> ("data"=w177:dbl)  [unwired: 1 in, 1 out]
    n195 = xnode "Database Variant To Data"("database variant"=w266, "type"=w263) -> ("data"=w176:dbl)  [unwired: 1 in, 1 out]
    n196 = xnode "Database Variant To Data"("database variant"=w267, "type"=w263) -> ("data"=w175:dbl)  [unwired: 1 in, 1 out]
    n197 = xnode "Database Variant To Data"("database variant"=w265, "type"=w262) -> ("data"=w248:i8)  [unwired: 1 in, 1 out]
    n198 = xnode "Database Variant To Data"("database variant"=w264, "type"=w262) -> ("data"=w247:i8)  [unwired: 1 in, 1 out]
    n199 = xnode "Database Variant To Data"("database variant"=w254, "type"=0.0) -> ("data"=w149:dbl)  [unwired: 1 in, 1 out]
    n200 = Multiply(x=w151, y=0.001) -> (x*y=w148:dbl)
    n201 = Build Array(w179, w180) -> (w251:dbl[])
    n202 = Add(x=w149, y=w148) -> (x+y=w147:dbl)
    "Peletron (MV)" <- w147
    n203 = Build Array(w178, w177) -> (w250:dbl[])
    n204 = Build Array(w176, w175) -> (w249:dbl[])
    n205 = Equal To 0?(x="Delay Ring") -> (x = 0?=w174:bool)
    n206 = xnode "Read/Write Control"("FPGA VI Reference In"=w216, "error in"=w215) -> ("Not Armed?"=w214:bool, "Del Not Armed?"=w168:bool)  [unwired: 2 out]
    n207 = local read "Delay Value"() -> (w173:dbl)
    n208 = call "calc_variables.vi"("var2"=w247, "Peletron"=w147, "var1"=w248, "Mass"=w249, "Charge"=w250, "Velocity"=w251) -> ("Mass out"=w240:dbl[], "Charge out"=w243:dbl[], "Velocity out"=w246:dbl[])  [unwired: 3 in]
    n209 = property on="Rearm Trigger" class="Bool (strict)"(error in=w215, "Value"=FALSE ("Rearm Trigger")) -> ()  [unwired: 1 in, 2 out]
    n210 = Divide(x="Delay Ring", y=0.93) -> (x/y=w212:dbl)
    n211 = Not(x=w214) -> (.not. x?=→"Armed":bool)
    n212 = Not(x=w168) -> (.not. x?=→"Del Armed":bool)
    n213 = Select(t=w173, s=w174, f=w212) -> (s? t:f=w211:dbl)
    n214 = And(x=w174, y=w169) -> (x .and. y?=w170:bool)
    n215 = property on="Peletron (MV)" class="DigNum (strict)"() -> ("Value"=w252:dbl)  [unwired: 2 in, 2 out]
    n216 = case shown="True" w170 {
      selector: w170 -> [w359 _]
      tunnel: w173 -> [_ w361]
      tunnel: [w359 w360] -> w171
      frame False {
      }
      frame True {
        n217 = call-poly <userlib>:"Data Changed__ogtk.vi"("DBL"=w361) -> ("Changed"=w360:bool)
      }
    }
    n218 = To Fixed-Point(number=w211) -> (fixed-point=w225:fxp<+,16,7>)  [unwired: 1 in]
    n219 = Index Array(array=w243, index #1=0 ("index"), index #2=1 ("index")) -> (element #1=w235:dbl, element #2=w234:dbl)
    "High Charge Limit (fC)" <- w234
    "Low Charge Limit (fC)" <- w235
    n220 = Index Array(array=w246, index #1=0 ("index"), index #2=1 ("index")) -> (element #1=w237:dbl, element #2=w236:dbl)
    "High Velocity" <- w236
    "Low Velocity" <- w237
    n221 = Index Array(array=w240, index #1=0 ("index"), index #2=1 ("index")) -> (element #1=w233:dbl, element #2=w232:dbl)
    "Low Mass (kg)" <- w233
    "High Mass (kg)" <- w232
    n222 = Bundle("Numeric"=w237, "Numeric"=w236, "Numeric"=w235, "Numeric"=w234, "Numeric"=w233, "Numeric"=w232, w229, 3333333.333, "Value"=w252, w225, w169) -> (w293:T7)  [unwired: 1 in]
    n223 = call "process_limits.vi"("old output cluster"=w300, "Input cluster"=w293) -> ("Update FPGA"=w228:bool, "output cluster"=w301:T8)  [unwired: 8 in]
    n224 = Unbundle By Name(w301) -> ("Low Velocity Count"=w289:i32, "High Velocity Count"=w288:i32, "Low Charge Limit (ADC ticks)"=w286:i16, "High Charge Limit (ADC ticks)"=w287:i16, "Low Mass (ADC*cycle^2)"=w291:i64, "High Mass (ADC*cycle^2)"=w292:i64, "Mult"=w224:fxp<+,16,7>)
    "Low velocity count" <- w289
    "High velocity count" <- w288
    "High Charge Limit" <- w287
    "Low Charge Limit" <- w286
    "High Mass Limit" <- w292
    "Low Mass Limit" <- w291
    n225 = Or(x=w228, y=w205) -> (x .or. y?=w210:bool)
    n226 = Or(x="Raise Threshold", y="Lower Threshold") -> (x .or. y?=w181:bool)
    n227 = Or(x=w181, y=w210) -> (x .or. y?=w182:bool)
    n228 = Build Array("Filter1 Threshold", "Filter2 Threshold", "Filter3 Threshold", "Filter4 Threshold", "Filter5 Threshold", "Filter6 Threshold", "Filter7 Threshold") -> (w165:i32[])
    n229 = case shown="True" "Lower Threshold" {
      tunnel: w165 -> [w362 w373]
      tunnel: w166 -> [_ w372]
      tunnel: [w362 w363] -> w195
      frame False {
      }
      frame True {
        n230 = Add(x=w373, y=w372) -> (x+y=w363:i32[])
        n231 = local write "Lower Threshold"(FALSE ("Lower Threshold")) -> ()
        n232 = Index Array(array=w363) -> (element #1=w370:i32, element #2=w369:i32, element #3=w368:i32, element #4=w367:i32, element #5=w366:i32, element #6=w365:i32, element #7=w364:i32)  [unwired: 7 in]
        n233 = local write "Filter1 Threshold"(w370) -> ()
        n234 = local write "Filter2 Threshold"(w369) -> ()
        n235 = local write "Filter3 Threshold"(w368) -> ()
        n236 = local write "Filter4 Threshold"(w367) -> ()
        n237 = local write "Filter5 Threshold"(w366) -> ()
        n238 = local write "Filter6 Threshold"(w365) -> ()
        n239 = local write "Filter7 Threshold"(w364) -> ()
      }
    }
    n240 = Or(x=w182, y=w171) -> (x .or. y?=w172:bool)
    "Updating FPGA" <- w172
    n241 = case shown="True" "Raise Threshold" {
      tunnel: w165 -> [_ w384]
      tunnel: w166 -> [_ w374]
      frame False {
      }
      frame True {
        n242 = Subtract(x=w384, y=w374) -> (x-y=w375:i32[])
        n243 = local write "Raise Threshold"(FALSE ("Raise Threshold")) -> ()
        n244 = Index Array(array=w375) -> (element #1=w382:i32, element #2=w381:i32, element #3=w380:i32, element #4=w379:i32, element #5=w378:i32, element #6=w377:i32, element #7=w376:i32)  [unwired: 7 in]
        n245 = local write "Filter1 Threshold"(w382) -> ()
        n246 = local write "Filter2 Threshold"(w381) -> ()
        n247 = local write "Filter3 Threshold"(w380) -> ()
        n248 = local write "Filter4 Threshold"(w379) -> ()
        n249 = local write "Filter5 Threshold"(w378) -> ()
        n250 = local write "Filter6 Threshold"(w377) -> ()
        n251 = local write "Filter7 Threshold"(w376) -> ()
      }
    }
    n252 = Index Array(array=w195) -> (element #1=w198:i32, element #2=w196:i32, element #3=w193:i32, element #4=w191:i32, element #5=w189:i32, element #6=w187:i32, element #7=w185:i32)  [unwired: 7 in]
    n253 = case shown="True" w172 {
      tunnel: w223 -> [w431 w459]
      tunnel: w222 -> [w432 w458]
      tunnel: [w431 w457] -> w322
      tunnel: [w432 w456] -> w321
      tunnel: w198 -> [_ w455]
      tunnel: w196 -> [_ w454]
      tunnel: w193 -> [_ w453]
      tunnel: w191 -> [_ w452]
      tunnel: w189 -> [_ w451]
      tunnel: w187 -> [_ w450]
      tunnel: w185 -> [_ w449]
      tunnel: [w430 w435] -> w298
      tunnel: w292 -> [_ w441]
      tunnel: w291 -> [_ w440]
      tunnel: w289 -> [_ w439]
      tunnel: w288 -> [_ w438]
      tunnel: w287 -> [_ w437]
      tunnel: w286 -> [_ w436]
      tunnel: w299 -> [w430 _]
      tunnel: w224 -> [_ w433]
      frame False {
      }
      frame True {
        n254 = xnode "Read/Write Control"("FPGA VI Reference In"=w459, "error in"=w458, "Low Velocity Count"=w439, "High Velocity Count"=w438, "Filter 1 threshold"=w455, "Filter 2 threshold"=w454, "Filter 3 threshold"=w453, "Filter 4 threshold"=w452, "Filter 5 threshold"=w451, "Filter 6 threshold"=w450, "Filter 7 threshold"=w449, "High Charge Limit"=w437, "Low Charge Limit"=w436, "High Mass Limit"=w441, "Low Mass Limit"=w440, "Mult1"=w433) -> ("FPGA VI Reference Out"=w457:refnum<k20>, "error out"=w456:errorcluster, "Filter 1 Detector 3 Correlation"=w448:i32, "Filter 2 Detector 3 Correlation"=w447:i32, "Filter 3 Detector 3 Correlation"=w446:i32, "Filter 4 Detector 3 Correlation"=w445:i32, "Filter 5 Detector 3 Correlation"=w444:i32, "Filter 6 Detector 3 Correlation"=w443:i32, "Filter 7 Detector 3 Correlation"=w442:i32)
        n255 = Get Date/Time In Seconds() -> (seconds since 1Jan1904=→"Last Update:":timestamp)
        n256 = Bundle("Filter 1 Detector 3 Correlation"=w448, "Filter 2 Detector 3 Correlation"=w447, "Filter 3 Detector 3 Correlation"=w446, "Filter 4 Detector 3 Correlation"=w445, "Filter 5 Detector 3 Correlation"=w444, "Filter 6 Detector 3 Correlation"=w443, "Filter 7 Detector 3 Correlation"=w442) -> (w435:T9)  [unwired: 1 in]
      }
    }
    n257 = call "filter_peaks.vi"("Correlation cluster"=w298, "Filter peak cluster"=w294, "Zero out"="Zero Peak Values", "Run Mode"="Run Mode") -> ("Blinking"=w285:bool, "status"=w290:T2, "Filter peak output"=w295:T4)  [unwired: 5 in]
    n258 = shared-variable "My Computer\\Network Shared Variables.lvlib\\FPGA Trigger"() -> ()  [unwired: 1 in, 2 out]
    n259 = Unbundle By Name(w295) -> ("Filter 1 Peak"=w319:i32, "Filter 2 Peak"=w318:i32, "Filter 3 Peak"=w317:i32, "Filter 4 Peak"=w316:i32, "Filter 5 Peak"=w315:i32, "Filter 6 Peak"=w314:i32, "Filter 7 Peak"=w313:i32)
    "Filter 1 Peak" <- w319
    "Filter 2 Peak" <- w318
    "Filter 3 Peak" <- w317
    "Filter 4 Peak" <- w316
    "Filter 5 Peak" <- w315
    "Filter 6 Peak" <- w314
    "Filter 7 Peak" <- w313
    n260 = property on="Filter 3 Peak" class="DigNum (strict)"("DisabledEnum"=w290, "Blinking"=w285) -> ()  [unwired: 2 in, 2 out]
    n261 = property on="Filter 4 Peak" class="DigNum (strict)"("DisabledEnum"=w290, "Blinking"=w285) -> ()  [unwired: 2 in, 2 out]
    n262 = property on="Filter 7 Peak" class="DigNum (strict)"("DisabledEnum"=w290, "Blinking"=w285) -> ()  [unwired: 2 in, 2 out]
    n263 = property on="Filter 5 Peak" class="DigNum (strict)"("DisabledEnum"=w290, "Blinking"=w285) -> ()  [unwired: 2 in, 2 out]
    n264 = property on="Filter 6 Peak" class="DigNum (strict)"("DisabledEnum"=w290, "Blinking"=w285) -> ()  [unwired: 2 in, 2 out]
    n265 = property on="Filter 2 Peak" class="DigNum (strict)"("DisabledEnum"=w290, "Blinking"=w285) -> ()  [unwired: 2 in, 2 out]
    n266 = property on="Filter 1 Peak" class="DigNum (strict)"("DisabledEnum"=w290, "Blinking"=w285) -> ()  [unwired: 2 in, 2 out]
    n267 = local read "Update Threshold"() -> (w201:bool)
    n268 = call-poly <userlib>:"Data Changed__ogtk.vi"("Boolean"=w201) -> ("Changed"=w202:bool)
    n269 = And(x=w202, y=w201) -> (x .and. y?=w200:bool)
    n270 = case shown="True" w200 {
      frame False {
      }
      frame True {
        n271 = local write "Update Threshold"(FALSE ("Update Threshold")) -> ()
      }
    }
    n272 = Or(x=w204, y=w201) -> (x .or. y?=w203:bool)
    "Sensitivity" <- w229
  }
  n273 = while {
    stop <- w749 stop-if-true
    n274 = case shown="True" "Rate Limiting" {
      frame False {
        n275 = property on="Rearm Trigger" class="Bool (strict)"("DisabledEnum"=T2."Enabled" ("Disabled")) -> ()  [unwired: 2 in, 2 out]
        n276 = property on="One Shot Mode" class="Bool (strict)"("DisabledEnum"=T2."Enabled" ("Disabled")) -> ()  [unwired: 2 in, 2 out]
      }
      frame True {
        n277 = local read "Armed"() -> (w753:bool)
        n278 = Get Date/Time In Seconds() -> (seconds since 1Jan1904=w752:timestamp)
        n279 = property on="Rearm Trigger" class="Bool (strict)"("DisabledEnum"=T2."Disabled and Grayed Out" ("Disabled")) -> ()  [unwired: 2 in, 2 out]
        n280 = case shown="False" w753 {
          tunnel: [w760 FALSE] -> w757
          tunnel: w752 -> [w759 _]
          frame False {
            n281 = flat-sequence {
              tunnel: w759 -> [w761]
              tunnel: [w761] -> w758
              tunnel: [TRUE] -> w760
              tunnel: w758 -> [w767]
              frame #0 {
                n282 = Multiply(x="Min. Time\nBetween Shots (s)", y=1000.0) -> (x*y=w764:dbl)
                n283 = Round Toward +Infinity(x=w764) -> (ceil(x): smallest int >= x=w762:dbl)
                n284 = Wait (ms)(milliseconds to wait=w762) -> ()  [unwired: 1 out]
              }
              frame #1 {
                n285 = Get Date/Time In Seconds() -> (seconds since 1Jan1904=w768:timestamp)
                n286 = Subtract(x=w768, y=w767) -> (x-y=→"Time Betwee Shots":dbl)
              }
            }
          }
          frame True {
          }
        }
        n287 = property on="One Shot Mode" class="Bool (strict)"("DisabledEnum"=T2."Disabled and Grayed Out" ("Disabled"), "Value"=TRUE ("One Shot Mode")) -> ()  [unwired: 2 in, 2 out]
        n288 = local write "Rearm Trigger"(w757) -> ()
      }
    }
    n289 = property on="stopping" class="Bool (strict)"() -> ("Value"=w749:bool)  [unwired: 2 in, 2 out]
  }
  n290 = call "connect out.vi"("error in (no error)"=w40, "connection reference"=w42) -> ()  [unwired: 9 in, 1 out]
  n291 = xnode "Close FPGA VI Reference"("FPGA VI Reference In"=w66, "error in"=w65) -> ("error out"=w68:errorcluster)
  n292 = call <vilib>:"General Error Handler.vi"("error in (no error)"=w68) -> ()  [unwired: 10 in, 5 out]
